vi "initialize python session.vi"(8 "error in (no error)":errorcluster, 10 "Optional Path to Python.exe":path=path "", 11 "Channel in":refnum<class "Channel.lvclass">) -> (0 "error out":errorcluster, 3 "Channel out":refnum<class "Channel.lvclass">)   [LabVIEW 2018, in "Channel.lvclass"]
uses:
  Channel.lvclass
  Channel.lvclass/Channel.ctl
  Save Image/Save Image.lvclass
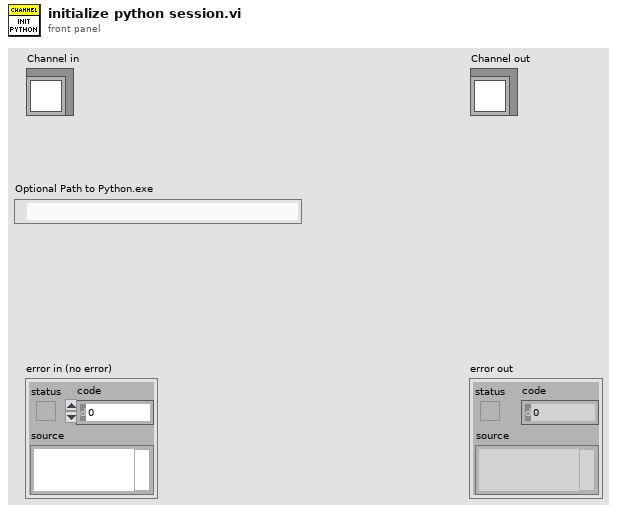
[diagram p1: front panel]
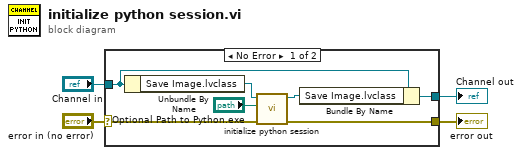
[diagram p0: block diagram]
diagram:
  n1 = case shown="No Error" "error in (no error)" {
    selector: "error in (no error)" -> [w6 w13]
    tunnel: [w7 w13] -> w3
    tunnel: [w11 w12] -> w1
    tunnel: "Channel in" -> [w10 w12]
    frame No Error {
      n2 = Unbundle By Name(w10) -> ("Save Image.lvclass"=w9:refnum<class "Save Image.lvclass">)
      n3 = call "initialize python session.vi"("error in (no error)"=w6, "Optional Path to Python.exe"="Optional Path to Python.exe", "Save Image in"=w9) -> ("error out"=w7:errorcluster, "Save Image out"=w8:refnum<class "Save Image.lvclass">)  [unwired: 7 in]
      n4 = Bundle By Name(cluster=w10, "Save Image.lvclass"=w8) -> (w11:refnum<class "Channel.lvclass">)
    }
    frame Error {
    }
  }
  "error out" <- w3
  "Channel out" <- w1
